vi "SpecAn Trace Type Set.vi"(0 "VISA In":refnum<visa-resource-name>, 5 "Error In":errorcluster, 6 "Trace":i32(ring)=1 items=["Trace 1"=1, "Trace 2"=2, "Trace 3"=3, "Trace 4"=4, "Trace 5"=5, "Trace 6"=6], 8 "Trace Type":i32(ring) items=["Clear Write", "Average", "Maximum Hold", "Minimum Hold"], 10 "Enable Trace Update (F: Disable)":bool=TRUE, 12 "Enable Trace Display (F: Disable)":bool=TRUE) -> (14 "VISA Out":refnum<visa-resource-name>, 19 "Error Out":errorcluster)   [LabVIEW 2015]
uses:
  Controls/FGV Action SpecAn Model.ctl
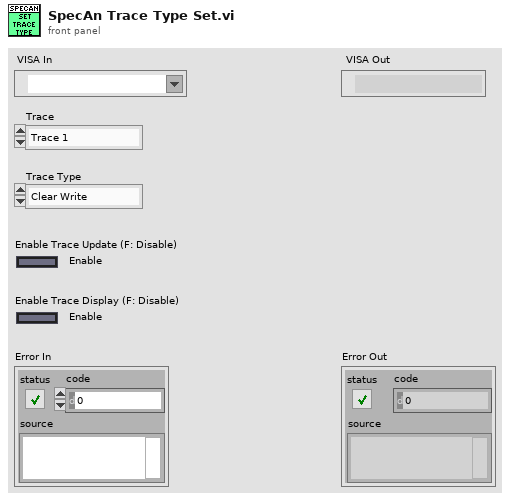
[diagram p1: front panel]
types:
  T1 = typedef "FGV Action SpecAn Model.ctl" = enum16{"Get", "Set"}
  T2 = typedef "SpecAn Model.ctl" = enum16{"E4440", "N9030"}
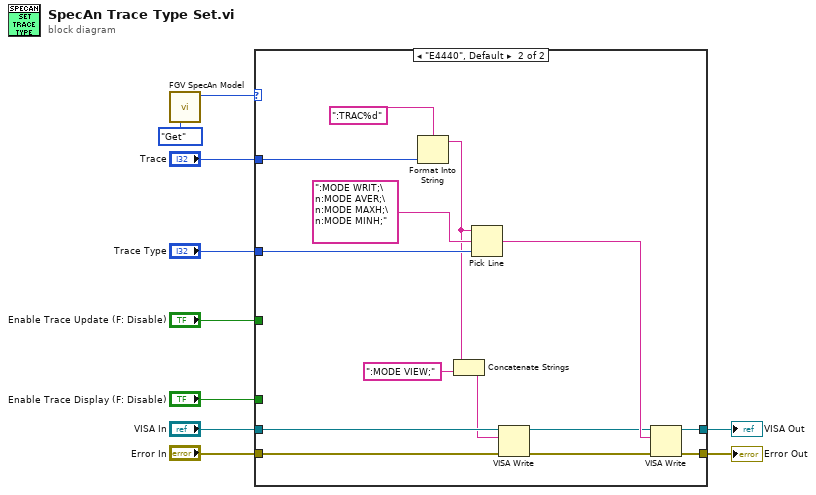
[diagram p0: block diagram]
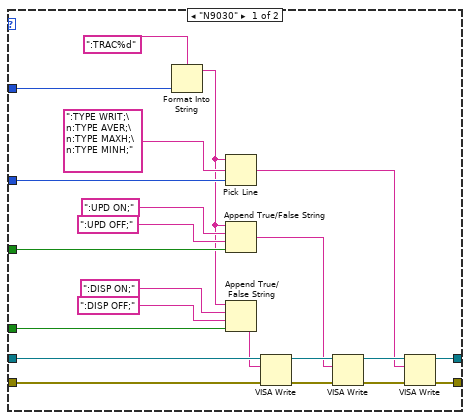
[diagram p2: hidden frame]
diagram:
  n1 = call "FGV SpecAn Model.vi"("Action"=FGV_Action_SpecAn_Model."Get") -> ("SA Model"=w1:T2)  [unwired: 6 in, 1 out]
  n2 = case shown="\"E4440\", Default" w1 {
    tunnel: "VISA In" -> [w32 w46]
    tunnel: "Error In" -> [w31 w45]
    tunnel: "Trace" -> [w28 w42]
    tunnel: "Trace Type" -> [w27 w41]
    tunnel: "Enable Trace Update (F: Disable)" -> [w24 _]
    tunnel: "Enable Trace Display (F: Disable)" -> [w23 _]
    tunnel: [w15 w40] -> w4
    tunnel: [w14 w39] -> w3
    frame "N9030" {
      n3 = Format Into String(format string=":TRAC%d" ("string (\"\")"), w28) -> (resulting string=w20:string)  [unwired: 2 in, 1 out]
      n4 = Pick Line(string ("")=w20, multi-line string=":TYPE WRIT;\n:TYPE AVER;\n:TYPE MAXH;\n:TYPE MINH;", line index=w27) -> (output string=w11:string)
      n5 = Append True/False String(1:w24, 2:":UPD OFF;" ("string"), 3:":UPD ON;" ("string"), 4:w20) -> (0:w12:string)
      n6 = Append True/False String(1:w23, 2:":DISP OFF;" ("string"), 3:":DISP ON;" ("string"), 4:w20) -> (0:w19:string)
      n7 = VISA Write(VISA resource name=w32, write buffer=w19, error in (no error)=w31) -> (VISA resource name out=w17:refnum<visa-resource-name>, error out=w18:errorcluster)  [unwired: 1 out]
      n8 = VISA Write(VISA resource name=w17, write buffer=w12, error in (no error)=w18) -> (VISA resource name out=w16:refnum<visa-resource-name>, error out=w13:errorcluster)  [unwired: 1 out]
      n9 = VISA Write(VISA resource name=w16, write buffer=w11, error in (no error)=w13) -> (VISA resource name out=w15:refnum<visa-resource-name>, error out=w14:errorcluster)  [unwired: 1 out]
    }
    frame "E4440", Default {
      n10 = Format Into String(format string=":TRAC%d" ("string (\"\")"), w42) -> (resulting string=w37:string)  [unwired: 2 in, 1 out]
      n11 = Concatenate Strings(w37, ":MODE VIEW;" ("string (\"\")")) -> (w35:string)
      n12 = Pick Line(string ("")=w37, multi-line string=":MODE WRIT;\n:MODE AVER;\n:MODE MAXH;\n:MODE MINH;", line index=w41) -> (output string=w38:string)
      n13 = VISA Write(VISA resource name=w46, write buffer=w35, error in (no error)=w45) -> (VISA resource name out=w33:refnum<visa-resource-name>, error out=w34:errorcluster)  [unwired: 1 out]
      n14 = VISA Write(VISA resource name=w33, write buffer=w38, error in (no error)=w34) -> (VISA resource name out=w40:refnum<visa-resource-name>, error out=w39:errorcluster)  [unwired: 1 out]
    }
  }
  "Error Out" <- w3
  "VISA Out" <- w4
